vi "Save_experiment.vi"(1 "Experiment parameters":T1={"Stimulus signal"={"Effector"="On-screen signal", "Delay"=-100.0}, "Reward period signal"={"Effector"="On-screen signal", "Delay"=0.0}, "Reward"={"Effector"="On-screen signal", "Condition"="In window", "Delay"=100.0}, "Response"={"Source"="Keyboard", "Window start"=0.0, "Threshold"=1, "Window duration"=250.0}, "Punishment"={"Effector"="On-screen signal", "Condition"="Wrong response"}}, 2 "Protocol File Path":path) -> ()   [LabVIEW 2016]
uses:
  <vilib>/Utility/xml.llb/Write to XML File(string).vi
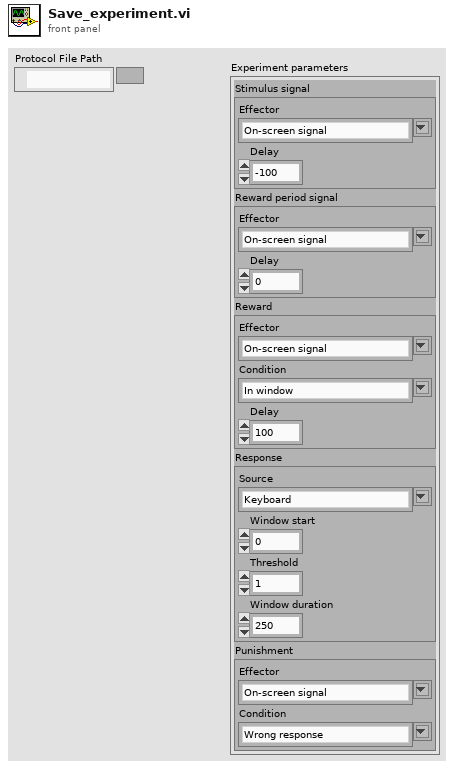
[diagram p1: front panel]
types:
  T1 = cluster{"Stimulus signal":cluster{"Effector":string, "Delay":dbl}, "Reward period signal":cluster{"Effector":string, "Delay":dbl}, "Reward":cluster{"Effector":string, "Condition":string, "Delay":dbl}, "Response":cluster{"Source":string, "Window start":dbl, "Threshold":u32, "Window duration":dbl}, "Punishment":cluster{"Effector":string, "Condition":string}}
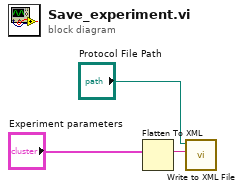
[diagram p0: block diagram]
diagram:
  n1 = Flatten To XML(anything="Experiment parameters") -> (xml string=w3:string)
  n2 = call-poly <vilib>:"Write to XML File.vi"("XML Input"=w3, "XML File Path"="Protocol File Path") -> ()  [unwired: 7 in, 3 out]
